vi "Write Best Cost.vi"(8 "error in (no error)":errorcluster, 10 "Best Cost":u64, 11 "State in":refnum<class "State.lvclass">) -> (0 "error out":errorcluster, 3 "State out":refnum<class "State.lvclass">)   [LabVIEW 2019, in "23.lvlib" / "State.lvclass"]
uses:
  State.lvclass
  C:/Users/craig.walker/Documents/GitHub/lv2019-LRU-Cache/LRU Node/LRU Node.lvclass
  lv2019-LRU-Cache/LRU Node/LRU Node.lvclass/LRU Node.ctl
  State Value/State Value.lvclass
  lv2019-LRU-Cache/LRU Node/LRU Node.lvclass
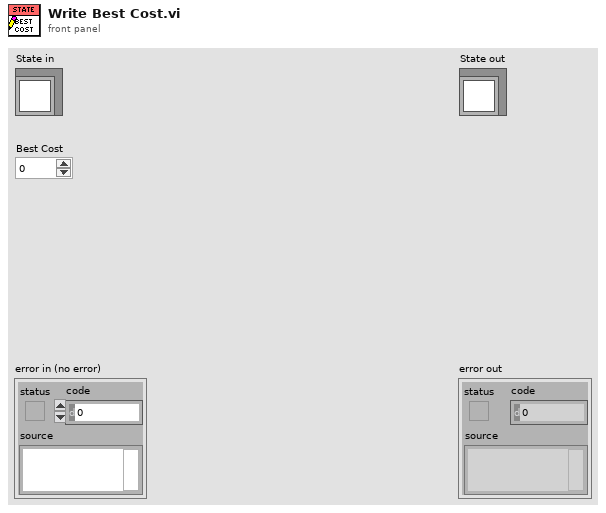
[diagram p1: front panel]
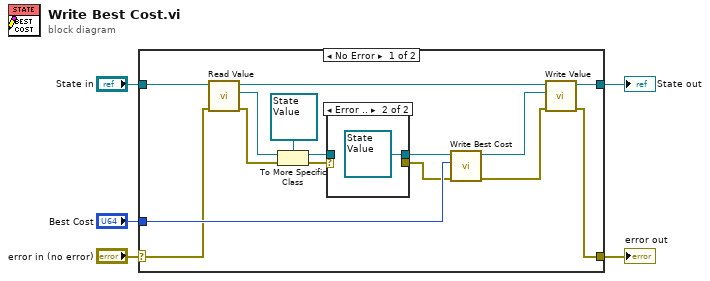
[diagram p0: block diagram]
diagram:
  n1 = case shown="No Error" "error in (no error)" {
    selector: "error in (no error)" -> [w11 w24]
    tunnel: [w10 w24] -> w4
    tunnel: [w15 w25] -> w2
    tunnel: "State in" -> [w19 w25]
    tunnel: "Best Cost" -> [w16 _]
    frame No Error {
      n2 = call "Read Value.vi"("error in (no error)"=w11, "LRU Node in"=w19) -> ("error out"=w13:errorcluster, "Value"=w18:refnum<class>, "LRU Node out"=w20:refnum<class "State.lvclass">)  [unwired: 7 in]
      n3 = To More Specific Class(target class=refnum<class "State Value.lvclass"> refnum ("State Value in"), reference=w18, error in=w13) -> (specific class reference=w8:refnum<class "State Value.lvclass">, error out=w9:errorcluster)
      n4 = case shown="Error .." w9 {
        selector: w9 -> [w21 _]
        tunnel: w8 -> [w22 _]
        tunnel: [w22 refnum<class "State Value.lvclass"> refnum ("State Value in")] -> w7
        tunnel: [w21 _] -> w6
        frame No Error {
        }
        frame Error {
        }
      }
      n5 = call-dynamic "Write Best Cost.vi"("error in (no error)"=w6, "Best Cost"=w16, "State Value in"=w7) -> ("error out"=w12:errorcluster, "State Value out"=w17:refnum<class "State Value.lvclass">)  [unwired: 7 in]
      n6 = call "Write Value.vi"("error in (no error)"=w12, "Value"=w17, "LRU Node in"=w20) -> ("error out"=w10:errorcluster, "LRU Node out"=w15:refnum<class "State.lvclass">)  [unwired: 7 in]
    }
    frame Error {
    }
  }
  "error out" <- w4
  "State out" <- w2
